vi "ShotInterception.vi"(6 "Ally?":bool, 8 "error in (no error)":errorcluster, 9 "Point":dbl[](array[numeric]), 10 "Game":refnum<class "Game.lvclass">, 11 "BallInterception in":refnum<class "BallInterception.lvclass">) -> (0 "error out":errorcluster, 2 "Evaluation":dbl, 3 "BallInterception out":refnum<class "BallInterception.lvclass">)   [LabVIEW 2023, in "BallInterception.lvclass"]
uses:
  BallInterception.lvclass
  Game_class/Game.lvclass
  Game_class/Game.lvclass/Game.ctl
  Referee_class/Referee.lvclass/Referee.ctl
  Team_class/Team.lvclass/Team.ctl
  Field_class/Field.lvclass/Field.ctl
  Robot_class/Robot.lvclass/Robot.ctl
  Object_class/Object.lvclass/Object.ctl
  <vilib>/Analysis/coordinate.llb/2D Cartesian Coordinate Shift (Scalar).vi
  <vilib>/Analysis/coordinate.llb/2D Cartesian Coordinate Rotation (Scalar).vi
  Robot_class/Read id.vi
  Object_class/Read position(x,y).vi
  Game_class/Read Referee.vi
  Game_class/Read EnemyRef.vi
  Game_class/Read BallRef.vi
  Game_class/Read Utilities.lvclass.vi
  Game_class/Read FieldRef.vi
  Field_class/Read enemyGoalPosition.vi
  Field_class/Read ourGoalPosition.vi
  Team_class/Read RobotRef.vi
  Referee_class/Read enemy_goalie_id.vi
  Enemy_class/Enemy.lvclass
  C:/Users/ebert/Documents/codes/SSL/repo/SSL_AI/Team_class/Team.lvclass
  Robot_class/Robot.lvclass
  C:/Users/ebert/Documents/codes/SSL/repo/SSL_AI/Object_class/Object.lvclass
  Referee_class/Referee.lvclass
  Ball_class/Ball.lvclass
  Utilities_class/Utilities.lvclass
  Field_class/Field.lvclass
  <vilib>/Analysis/NI_AALPro.lvlib
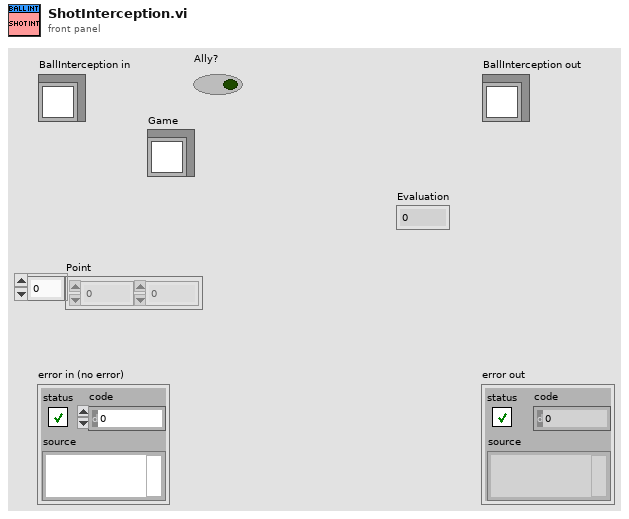
[diagram p1: front panel]
types:
  T1 = typedef "STPParameters.ctl" = cluster{"Skills":T2, "TestSkill":T4, "Events":cluster{"distanceToBallPossession":dbl, "timeForPossessionThreshold":dbl}, "Criteria":cluster{"OpenAngleToGoal":cluster{"minAngle":dbl, "maxAngle":dbl, "minEvaluation":dbl}, "PassDistance":cluster{"maxDistance":dbl, "minDistance":dbl}, "ShotTime":cluster{"shotSpeed":dbl, "keeperSpeed":dbl, "maxShotDistance":dbl, "minEvaluation":dbl}, "OneTouchShot":cluster{"MaxAngle":dbl, "minEvaluation":dbl}, "BallInterception":cluster{"minEnemySpeed":dbl, "maxEnemySpeed":dbl, "chipPassDistance":dbl, "chipPassEval":dbl, "minEvaluation":dbl}}, "minPassSpeed":dbl, "maxPassSpeed":dbl, "AllyTeamIds":T5[]}
  T2 = typedef "Skills.ctl" = cluster{"CirculateBall":T3, "ProtectBall":cluster{"DistanceFromBall":dbl}}
  T3 = typedef "CIrculateSkillParameters.ctl" = cluster{"rotationAngle":dbl, "velocityFactor":dbl, "OrientationFactor":dbl}
  T4 = typedef "TestSkills.ctl" = enum16{"AlignSkill", "PassSkill", "CirculateBall", "OneTouchShotSkill", "KickToSkill_v2", "ShootSkill", "InterceptBall", "Exit", "GoToSkill_v2"}
  T5 = typedef "AllyTeam.ctl" = enum16{"Keeper", "Defender", "Attacker"}
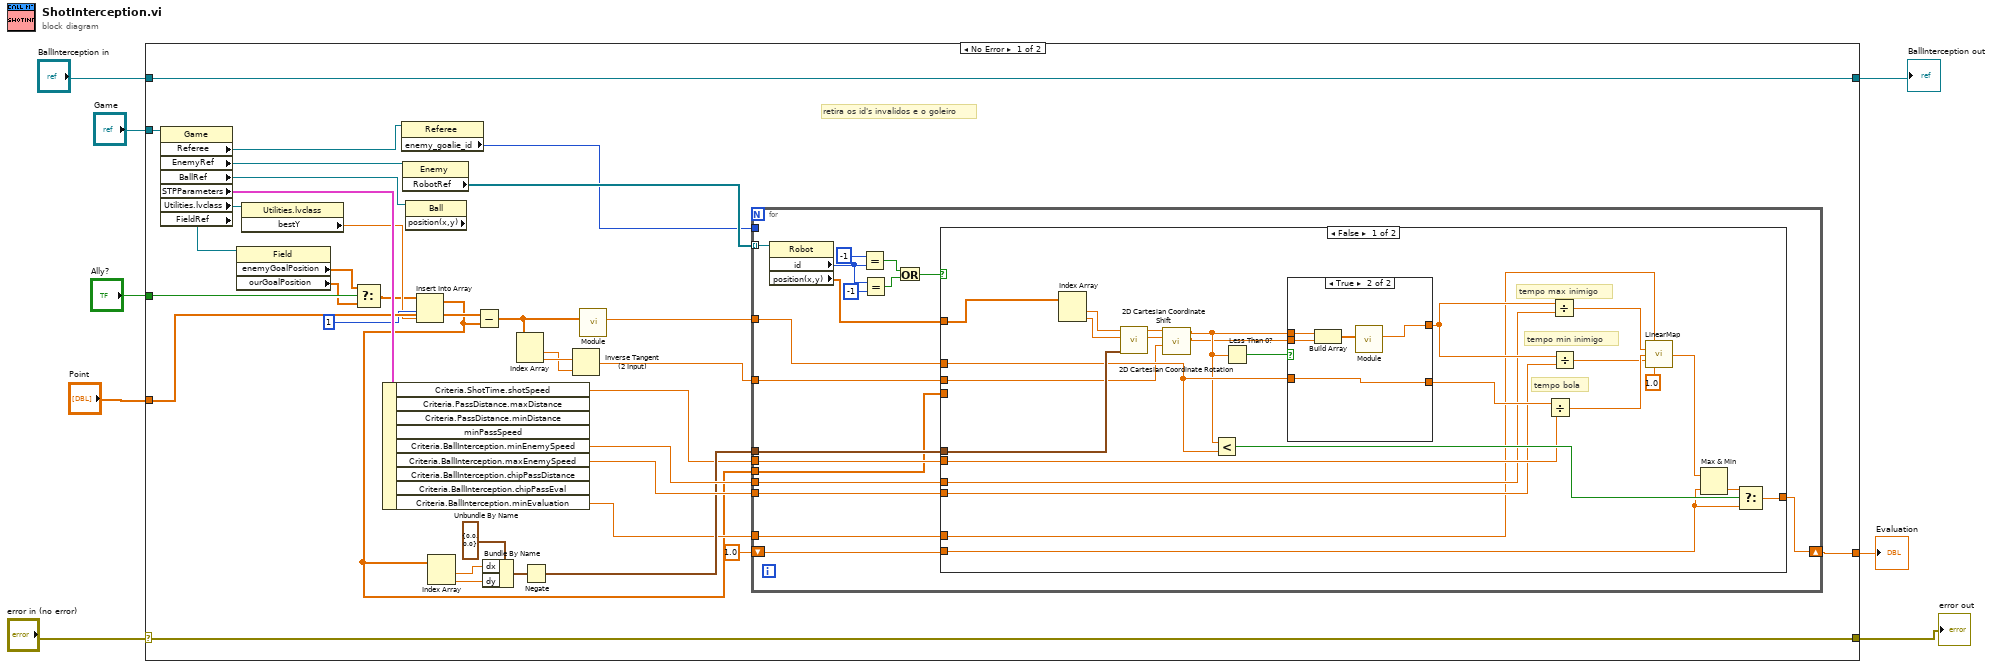
[diagram p0: block diagram]
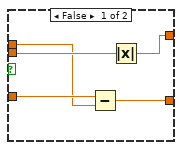
[diagram p2: hidden frame]
diagram:
  n1 = case shown="No Error" "error in (no error)" {
    selector: "error in (no error)" -> [w43 w100]
    tunnel: [w43 w100] -> w2
    tunnel: "BallInterception in" -> [w42 w99]
    tunnel: [w42 w99] -> w4
    tunnel: "Game" -> [w41 _]
    tunnel: "Point" -> [w18 _]
    tunnel: [w25 _] -> w6
    tunnel: "Ally?" -> [w12 _]
    frame No Error {
      # "retira os id's invalidos e o goleiro"
      n2 = property class="Game"(reference=w41) -> ("Referee"=w38:refnum<class "Referee.lvclass">, "EnemyRef"=w40:refnum<class "Enemy.lvclass">, "BallRef"=w36:refnum<class "Ball.lvclass">, "STPParameters"=w28:T1, "Utilities.lvclass"=w19:refnum<class "Utilities.lvclass">, "FieldRef"=w17:refnum<class "Field.lvclass">)  [unwired: 1 in, 2 out]
      n3 = property class="Field"(reference=w17) -> ("enemyGoalPosition"=w10:dbl[], "ourGoalPosition"=w9:dbl[])  [unwired: 1 in, 2 out]
      n4 = property class="Utilities.lvclass"(reference=w19) -> ("bestY"=w15:dbl)  [unwired: 1 in, 2 out]
      n5 = Select(t=w10, s=w12, f=w9) -> (s? t:f=w11:dbl[])
      n6 = Unbundle By Name(w28) -> ("Criteria.ShotTime.shotSpeed"=w13:dbl, "Criteria.BallInterception.minEnemySpeed"=w24:dbl, "Criteria.BallInterception.maxEnemySpeed"=w23:dbl, "Criteria.BallInterception.minEvaluation"=w20:dbl)  [unwired: 5 out]
      n7 = property class="Referee"(reference=w38) -> ("enemy_goalie_id"=w37:i32)  [unwired: 1 in, 2 out]
      n8 = property class="Enemy"(reference=w40) -> ("RobotRef"=w39:refnum<class "Robot.lvclass">[])  [unwired: 1 in, 2 out]
      n9 = property class="Ball" props=["position(x,y)"](reference=w36) -> ()  [unwired: 1 in, 3 out]
      n10 = Insert Into Array(array=w11, index=1, new element=w15) -> (w14:dbl[])
      n11 = Index Array(array=w14) -> (element #1=w31:dbl, element #2=w30:dbl)  [unwired: 2 in]
      n12 = Subtract(x=w18, y=w14) -> (x-y=w29:dbl[])
      n13 = Bundle By Name(cluster=cluster{"dx":dbl, "dy":dbl} {"dx"=0.0, "dy"=0.0} ("shift"), "dx"=w31, "dy"=w30) -> (w22:cluster{"dx":dbl, "dy":dbl})
      n14 = Index Array(array=w29) -> (element #1=w34:dbl, element #2=w35:dbl)  [unwired: 2 in]
      n15 = Negate(x=w22) -> (-x=w21:cluster{"dx":dbl, "dy":dbl})
      n16 = Inverse Tangent (2 Input)(1:w34, 2:w35) -> (0:w33:dbl)
      n17 = call "Module.vi"("2D vector"=w29) -> ("Modulo"=w27:dbl)  [unwired: 8 in, 2 out]
      n18 = for {
        tunnel: w39 -> [w60] mode=indexing
        tunnel: w37 -> [_]
        tunnel: w33 -> [w55]
        tunnel: w21 -> [w53]
        tunnel: w27 -> [w52]
        tunnel: w13 -> [w51]
        shift-right: [w49] -> w25
        shift-left: 1.0 ("Numeric") -> [w50]
        tunnel: w14 -> [w48]
        tunnel: w24 -> [w47]
        tunnel: w23 -> [w46]
        tunnel: w20 -> [w45]
        n19 = property class="Robot"(reference=w60) -> ("id"=w59:i32, "position(x,y)"=w54:dbl[])  [unwired: 1 in, 2 out]
        n20 = Equal?(x=-1, y=w59) -> (x = y?=w57:bool)
        n21 = Equal?(x=w59, y=-1) -> (x = y?=w56:bool)
        n22 = Or(x=w57, y=w56) -> (x .or. y?=w61:bool)
        n23 = case shown="False" w61 {
          tunnel: w55 -> [w69 _]
          tunnel: w54 -> [w83 _]
          tunnel: w53 -> [w87 _]
          tunnel: w52 -> [w78 _]
          tunnel: w51 -> [w79 _]
          tunnel: w50 -> [w70 w98]
          tunnel: [w84 w98] -> w49
          tunnel: w48 -> [_ _]
          tunnel: w47 -> [w76 _]
          tunnel: w46 -> [w75 _]
          tunnel: w45 -> [w62 _]
          frame False {
            # "tempo bola"
            # "tempo min inimigo"
            # "tempo max inimigo"
            n24 = Index Array(array=w83) -> (element #1=w68:dbl, element #2=w67:dbl)  [unwired: 2 in]
            n25 = call-poly <vilib>:"2D Cartesian Coordinate Shift.vi"("shift"=w87, "y"=w67, "x"=w68) -> ("y out"=w65:dbl, "x out"=w66:dbl)  [unwired: 6 in, 1 out]
            n26 = call-poly <vilib>:"2D Cartesian Coordinate Rotation.vi"("theta"=w69, "y"=w65, "x"=w66) -> ("y out"=w63:dbl, "x out"=w64:dbl)  [unwired: 6 in, 1 out]
            n27 = Less?(x=w64, y=w78) -> (x < y?=w85:bool)
            n28 = Less Than 0?(x=w64) -> (x < 0?=w86:bool)
            n29 = case shown="True" w86 {
              tunnel: w64 -> [w88 w95]
              tunnel: w63 -> [w91 w93]
              tunnel: [w90 w97] -> w80
              tunnel: w78 -> [w89 w96]
              tunnel: [w92 w96] -> w77
              frame False {
                n30 = Subtract(x=w89, y=w88) -> (x-y=w92:dbl)
                n31 = Absolute Value(x=w91) -> (abs(x)=w90:dbl)
              }
              frame True {
                n32 = Build Array(w95, w93) -> (w94:dbl[])
                n33 = call "Module.vi"("2D vector"=w94) -> ("Modulo"=w97:dbl)  [unwired: 8 in, 2 out]
              }
            }
            n34 = Divide(x=w77, y=w79) -> (x/y=w82:dbl)
            n35 = Divide(x=w80, y=w76) -> (x/y=w74:dbl)
            n36 = Divide(x=w80, y=w75) -> (x/y=w73:dbl)
            n37 = call "LinearMap.vi"("MaxY"=w62, "MaxX"=w74, "X"=w82, "MinX"=w73, "MinY"=1.0) -> ("Y"=w72:dbl)  [unwired: 8 in, 2 out]
            n38 = Max & Min(x=w72, y=w70) -> (min(x,y)=w71:dbl)  [unwired: 1 out]
            n39 = Select(t=w71, s=w85, f=w70) -> (s? t:f=w84:dbl)
          }
          frame True {
          }
        }
      }
    }
    frame Error {
    }
  }
  "error out" <- w2
  "BallInterception out" <- w4
  "Evaluation" <- w6
